vi "Dialog DISabilita potenza.vi"() -> (2 "DISABILITA":bool)   [LabVIEW 2019]
panel:
  in  "Annulla":bool
  in  "ABILITA POTENZA":bool
  # "APRIRE IL TELERUTTORE \n         DI POTENZA?"
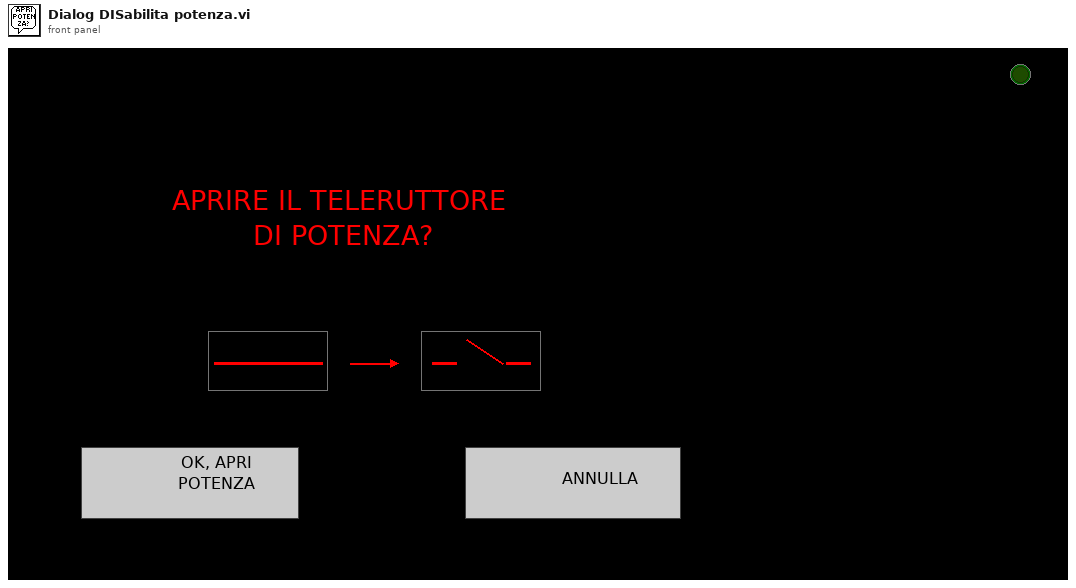
[diagram p1: front panel]
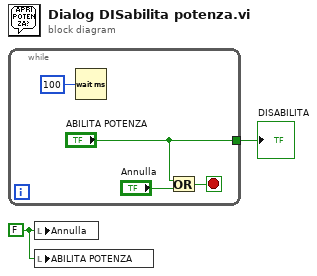
[diagram p0: block diagram]
diagram:
  w1 = FALSE
  n1 = while {
    tunnel: ["ABILITA POTENZA"] -> w2
    stop <- w5 stop-if-true
    n2 = Wait (ms)(milliseconds to wait=u32 100) -> ()  [unwired: 1 out]
    n3 = Or(x="ABILITA POTENZA", y="Annulla") -> (x .or. y?=w5:bool)
  }
  "DISABILITA" <- w2
  n4 = local write "Annulla"(w1) -> ()
  n5 = local write "ABILITA POTENZA"(w1) -> ()
